vi "initialize.vi"(8 "error in (no error)":errorcluster) -> (0 "error IO":errorcluster, 2 "pdbm_testsys_reg_event":T1, 3 "pdbm_testsys_event":T2)   [LabVIEW 2015, in "pdbm_test_system.lvlib"]
uses:
  pdbm_test_system.lvlib
  pdbm_testsys_taskroute_inter/UsrDefine/pdbm_testsys_reqst_data.ctl
  UsrDefine/pdbm_testsystem_feedback_data.ctl
  pdbm_testsys_taskroute_inter/pdbm_testsys_taskroute_inter.lvlib
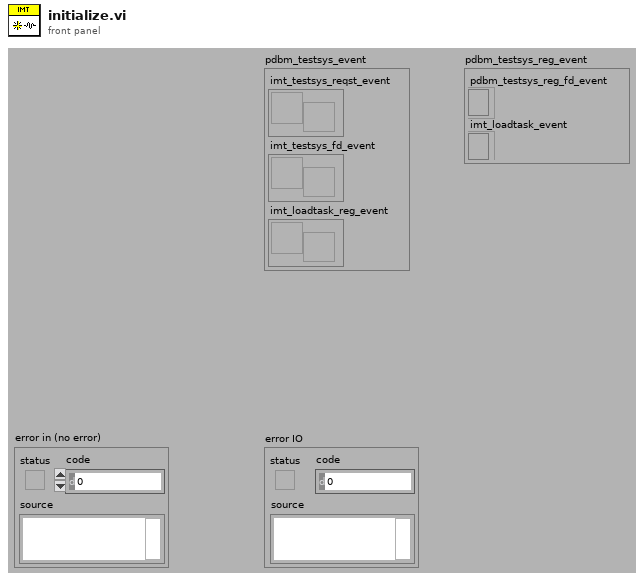
[diagram p1: front panel]
types:
  T1 = cluster{"pdbm_testsys_reg_fd_event":refnum<event-registration>, "imt_loadtask_event":refnum<event-registration>}
  T2 = cluster{"imt_testsys_reqst_event":refnum<user-event>, "imt_testsys_fd_event":refnum<user-event>, "imt_loadtask_reg_event":refnum<user-event>}
  T3 = cluster{"pdbm_testsys_reqst_event":refnum<user-event>, "pdbm_testsys_feedback_event":refnum<user-event>, "LoadTask":refnum<user-event>}
  T4 = cluster{"Event Registration Refnum":refnum<event-registration>, "Event Registration Refnum":refnum<event-registration>}
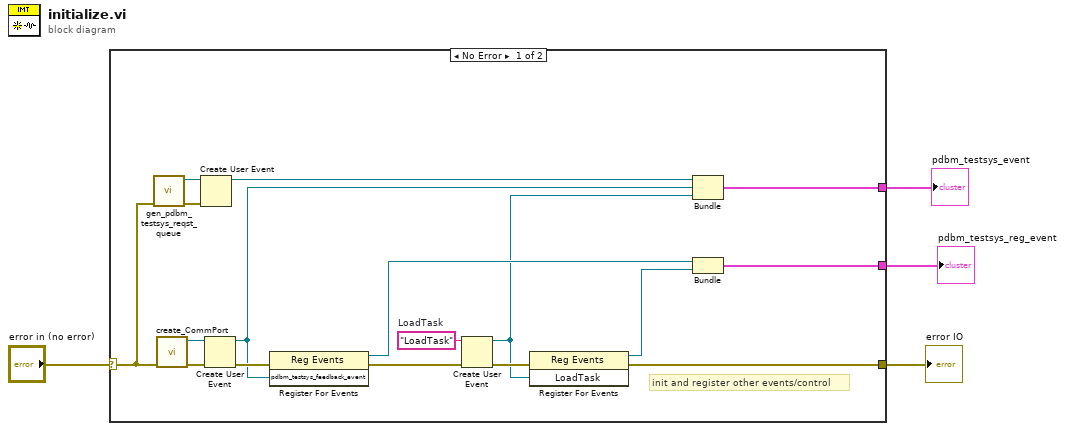
[diagram p0: block diagram]
diagram:
  n1 = case shown="No Error" "error in (no error)" {
    selector: "error in (no error)" -> [w18 w22]
    tunnel: [w7 w22] -> w3
    tunnel: [w13 _] -> w2
    tunnel: [w11 _] -> w1
    frame No Error {
      w9 = "LoadTask"  # LoadTask
      # "init and register other events/control"
      n2 = call "gen_pdbm_testsys_reqst_queue.vi"("error in (no error)"=w18) -> ("error IO"=w16:errorcluster, "pdbm_testsys_reqst_event"=w17:refnum<queue>)  [unwired: 9 in]
      n3 = call "create_CommPort.vi"("error in (no error)"=w18) -> ("error out"=w20:errorcluster, "pdbm_testsys_feedback_event"=w21:refnum<queue>)  [unwired: 9 in]
      n4 = Create User Event(user event datatype=w17, error in=w16) -> (user event=w15:refnum<user-event>)  [unwired: 1 out]
      n5 = Create User Event(user event datatype=w21, error in=w20) -> (user event=w14:refnum<user-event>, error out=w19:errorcluster)
      n6 = register-events(error in=w19, w14) -> (reference out=w12:refnum<event-registration>, error out=w10:errorcluster)  [unwired: 1 in]
      n7 = Create User Event(user event datatype=w9, error in=w10) -> (user event=w6:refnum<user-event>, error out=w8:errorcluster)
      n8 = register-events(error in=w8, w6) -> (reference out=w5:refnum<event-registration>, error out=w7:errorcluster)  [unwired: 1 in]
      n9 = Bundle("pdbm_testsys_reqst_event"=w15, "pdbm_testsys_feedback_event"=w14, "LoadTask"=w6) -> (w13:T3)  [unwired: 1 in]
      n10 = Bundle("Event Registration Refnum"=w12, "Event Registration Refnum"=w5) -> (w11:T4)  [unwired: 1 in]
    }
    frame Error {
    }
  }
  "error IO" <- w3
  "pdbm_testsys_event" <- w2
  "pdbm_testsys_reg_event" <- w1
